vi "ROS_Topic_Close_Primitive.vi"(3 "ROS in":T1={"topic port"=0, "Node"="", "topic"="", "type"="", "node port"=0, "error "={"status"=FALSE, "code"=0, "source"=""}, "Direction"=enum."Node", "Update (ms)"=1, "FIFO size"=1}) -> (0 "error out":errorcluster)   [LabVIEW 2014]
doc: "Closes a topic. If no topic is defined, it will close all topics and the node."
uses:
  <userlib>/ROS for LabVIEW Software.lnk/ROS/Code/SubVIs/_ROSControl.ctl
  <userlib>/ROS for LabVIEW Software.lnk/ROS/Code/SubVIs/_ROSDirection.ctl
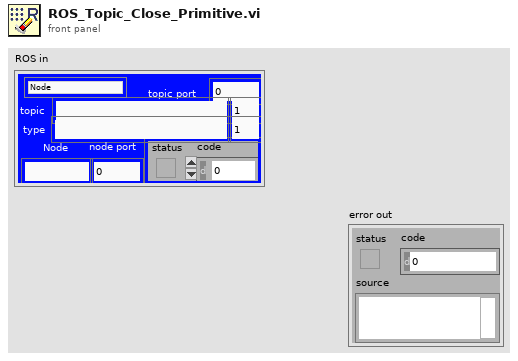
[diagram p1: front panel]
types:
  T1 = typedef "_ROSControl.ctl" = cluster{"topic port":u16, "Node":string, "topic":string, "type":string, "node port":u16, "error ":errorcluster, "Direction":T2, "Update (ms)":u16, "FIFO size":u16}
  T2 = typedef "_ROSDirection.ctl" = enum16{"Node", "Publisher", "Subscriber", "ServiceClient", "ServiceProvider"}
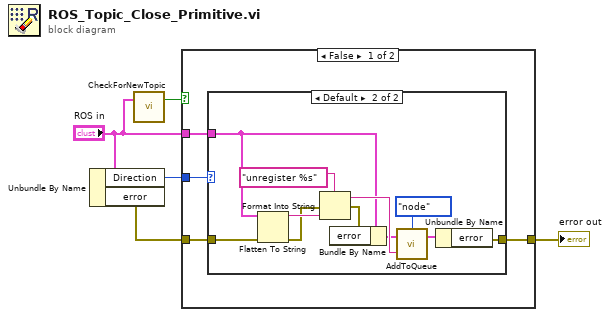
[diagram p0: block diagram]
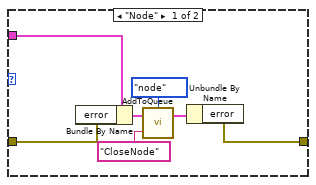
[diagram p2: hidden frame]
diagram:
  n1 = Unbundle By Name("ROS in") -> ("Direction"=w4:T2, "error"=w1:errorcluster)
  n2 = call <userlib>:"CheckForNewTopic.vi"("ROS"="ROS in") -> ("new?"=w2:bool)  [unwired: 2 in]
  n3 = case shown="False" w2 {
    tunnel: w1 -> [w9 w28]
    tunnel: [w8 w28] -> w5
    tunnel: w4 -> [w7 _]
    tunnel: "ROS in" -> [w6 _]
    frame False {
      n4 = case shown="Default" w7 {
        tunnel: w6 -> [w13 w21]
        tunnel: w9 -> [w14 w25]
        tunnel: [w10 w17] -> w8
        frame "Node" {
          n5 = Bundle By Name(cluster=w13, "error"=w14) -> (w12:T1)
          n6 = call <userlib>:"AddToQueue.vi"("Cmd"="CloseNode" ("format string"), "ROS"=w12, "Type"=enum16{"topic", "node"}."node" ("Name")) -> ("ROS out"=w11:T1)  [unwired: 2 in]
          n7 = Unbundle By Name(w11) -> ("error"=w10:errorcluster)
        }
        frame Default {
          n8 = Flatten To String(anything=w21, error in (no error)=w25) -> (data string=w26:string, error out=w22:errorcluster)  [unwired: 2 in, 1 out]
          n9 = Format Into String(format string="unregister %s", error in=w22, w26) -> (resulting string=w23:string, error out=w20:errorcluster)  [unwired: 1 in]
          n10 = Bundle By Name(cluster=w21, "error"=w20) -> (w19:T1)
          n11 = call <userlib>:"AddToQueue.vi"("Cmd"=w23, "ROS"=w19, "Type"=enum16{"topic", "node"}."node" ("Name")) -> ("ROS out"=w18:T1)  [unwired: 2 in]
          n12 = Unbundle By Name(w18) -> ("error"=w17:errorcluster)
        }
      }
    }
    frame True {
      # "If not in the list then never started"
    }
  }
  "error out" <- w5
